vi "Write Plot Area Colors.vi"(5 "Plot Area Colors":T1, 9 "GraphChart in":refnum<class "GraphChart.lvclass">) -> (3 "GraphChart out":refnum<class "GraphChart.lvclass">)   [LabVIEW 2014, in "Raspberry Pi Compatible Compiler for LabVIEW.lvlib" / "GraphChart.lvclass"]
uses:
  GraphChart.lvclass
  GraphChart.lvclass/GraphChart.ctl
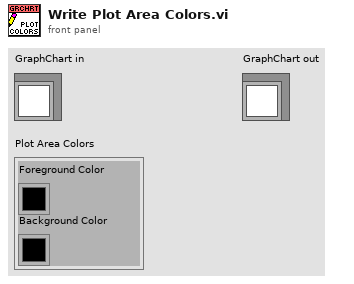
[diagram p1: front panel]
types:
  T1 = cluster{"Foreground Color":u32, "Background Color":u32}
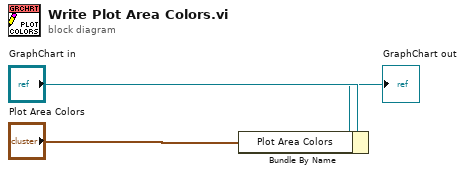
[diagram p0: block diagram]
diagram:
  n1 = Bundle By Name(cluster="GraphChart in", "Plot Area Colors"="Plot Area Colors") -> (→"GraphChart out":refnum<class "GraphChart.lvclass">)
